vi "Compress Jpeg.vi"(4 "pitch":i32, 5 "Chrominance Subsampling":T1(ring), 6 "Pixel Format":T2(ring), 7 "jpegQual":i32=80, 8 "error in (no error)":errorcluster, 9 "height":i32, 10 "width":i32, 11 "srcBuf":u8[](array[numeric])) -> (0 "error out":errorcluster, 3 "jpegImage":u8[](array[numeric]))   [LabVIEW 2020, in "LV Tiff.lvlib"]
uses:
  LV Tiff.lvlib
  x64/turbojpeg.dll
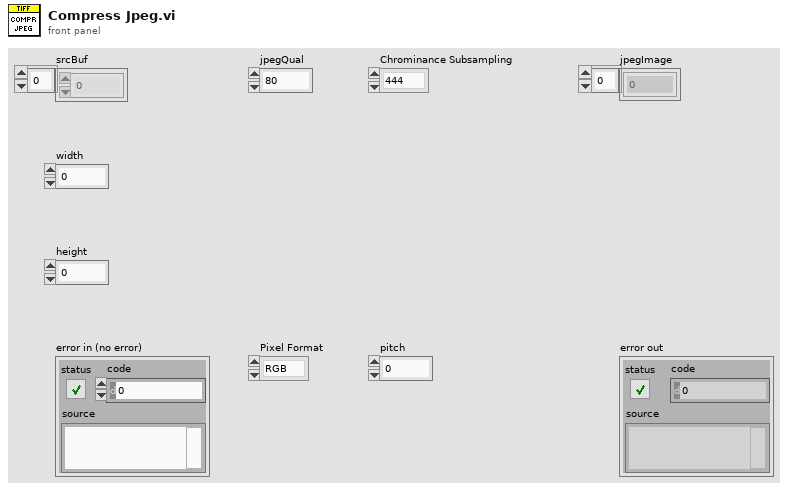
[diagram p1: front panel]
types:
  T1 = enum16{"444", "422", "420", "Gray", "440", "411"}
  T2 = enum16{"RGB", "BGR", "RGBX", "BGRX", "XBGR", "XRGB", "Gray", "RGBA", "BGRA", "ABGR", "ARGB", "CMYK"}
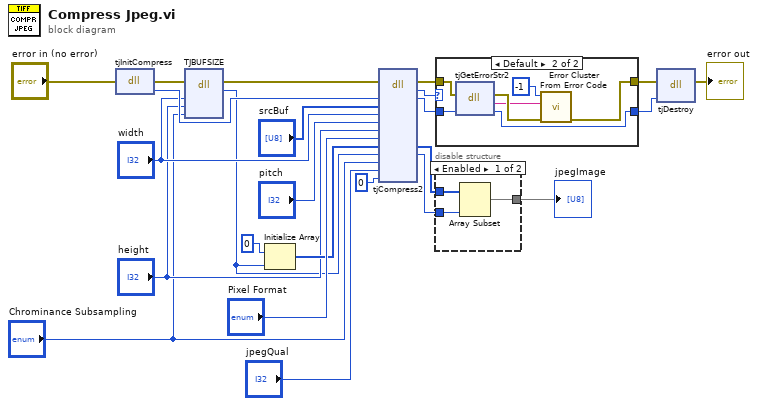
[diagram p0: block diagram]
diagram:
  n1 = dll-call lib="C:/Dev/Labview/Schmiedeteilvermessung/Source/libs/SK Utils/LV Tiff/_Helpers/x64/turbojpeg.dll" fn="tjInitCompress"(error in="error in (no error)") -> (error out=w15:errorcluster, "return type"=w24:i64)  [unwired: 2 in, 1 out]
  n2 = dll-call lib="C:/Dev/Labview/Schmiedeteilvermessung/Source/libs/SK Utils/LV Tiff/_Helpers/x64/turbojpeg.dll" fn="TJBUFSIZE"(error in=w15, "width"="width", "height"="height", "jpegSubsamp"="Chrominance Subsampling") -> (error out=w14:errorcluster, "return type"=w9:u32)  [unwired: 5 in, 1 out]
  n3 = Initialize Array(u8 0, w9) -> (w19:u8[])
  n4 = dll-call lib="C:/Dev/Labview/Schmiedeteilvermessung/Source/libs/SK Utils/LV Tiff/_Helpers/x64/turbojpeg.dll" fn="tjCompress2"(error in=w14, "handle"=w24, "srcBuf"="srcBuf", "width"="width", "pitch"="pitch", "height"="height", "pixelFormat"="Pixel Format", "jpegBuf"=w19, "jpegSize"=w9, "jpegSubsamp"="Chrominance Subsampling", "jpegQual"="jpegQual", "flags"=0) -> (error out=w7:errorcluster, "return type"=w3:i32, "handle"=w5:i64, "jpegBuf"=w13:u8[], "jpegSize"=w1:u32)  [unwired: 10 in, 1 out]
  n5 = case shown="Default" w3 {
    tunnel: w7 -> [w25 w33]
    tunnel: [w25 w29] -> w6
    tunnel: w5 -> [w26 w31]
    tunnel: [w26 w30] -> w4
    frame 0 {
    }
    frame Default {
      n6 = dll-call lib="C:/Dev/Labview/Schmiedeteilvermessung/Source/libs/SK Utils/LV Tiff/_Helpers/x64/turbojpeg.dll" fn="tjGetErrorStr2"(error in=w33, "handle"=w31) -> (error out=w32:errorcluster, "return type"=w27:string, "handle"=w30:i64)  [unwired: 2 in, 1 out]
      n7 = call <vilib>:"Error Cluster From Error Code.vi"("error in (no error)"=w32, "error message (\"\")"=w27, "error code (0)"=-1) -> ("error out"=w29:errorcluster)  [unwired: 6 in]
    }
  }
  n8 = disable-structure shown="Enabled" {
    disable-tunnel: w13 -> [w36 w37]
    disable-tunnel: w1 -> [w35 _]
    disable-tunnel: [w34 w37] -> w2
    frame Enabled {
      n9 = Array Subset(array=w36, length=w35) -> (w34:u8[])  [unwired: 1 in]
    }
    frame Disabled {
    }
  }
  "jpegImage" <- w2
  n10 = dll-call lib="C:/Dev/Labview/Schmiedeteilvermessung/Source/libs/SK Utils/LV Tiff/_Helpers/x64/turbojpeg.dll" fn="tjDestroy"(error in=w6, "handle"=w4) -> (error out=→"error out":errorcluster)  [unwired: 4 in, 1 out]
